vi "Write String.vi"(8 "error in (no error)":errorcluster, 9 "Colour":T1 items=["red"=0, "orange"=18, "yellow"=24, "green"=82, "cyan"=127, "blue"=170, "purple"=195, "pink"=220, "white"=254, "black"=255], 10 "String":string, 11 "Grove 2 RGB LED Matrix In":refnum<class "Grove 2 RGB LED Matrix.lvclass">) -> (0 "error out":errorcluster, 3 "Grove 2 RGB LED Matrix Out":refnum<class "Grove 2 RGB LED Matrix.lvclass">)   [LabVIEW 2020, in "CTI-Peripheral.lvlib" / "Grove 2 RGB LED Matrix.lvclass"]
uses:
  Grove 2 RGB LED Matrix.lvclass
  Data Types/Colors.ctl
  Data Types/MatrixI2CCommand.ctl
  Grove 2 RGB LED Matrix.lvclass/Grove 2 RGB LED Matrix.ctl
  CTI/I2C Connection/I2C Connection.lvclass/I2C Connection.ctl
  CTI/Session/I2C Write Data.vi
  CTI/I2C Connection/I2C Connection.lvclass
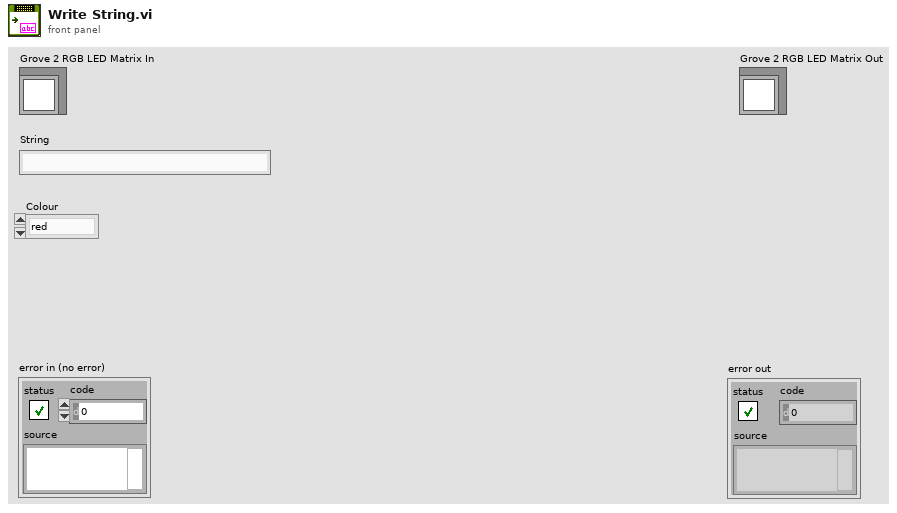
[diagram p1: front panel]
types:
  T1 = typedef "CTI-Peripheral.lvlib/Grove 2 RGB LED Matrix.lvclass/Colors.ctl" = u8
  T2 = typedef "CTI-Peripheral.lvlib/Grove 2 RGB LED Matrix.lvclass/MatrixI2CCommand.ctl" = u8
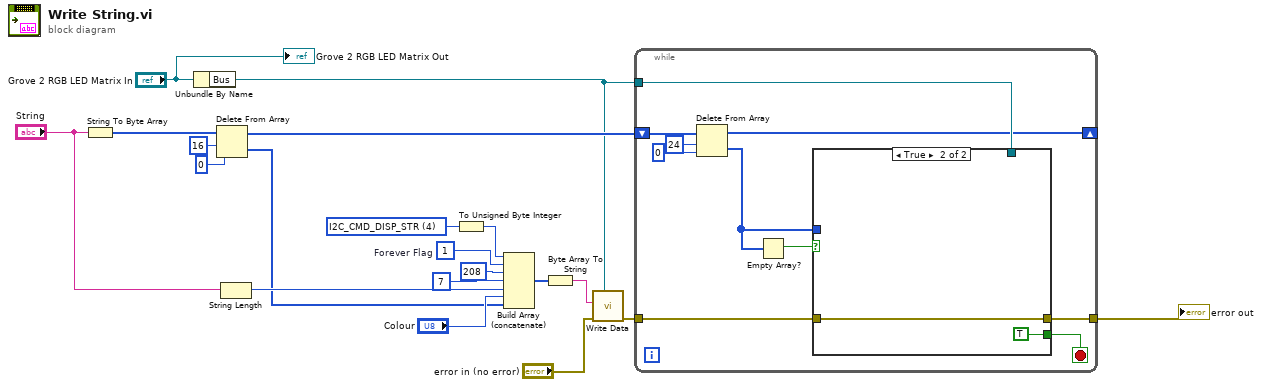
[diagram p0: block diagram]
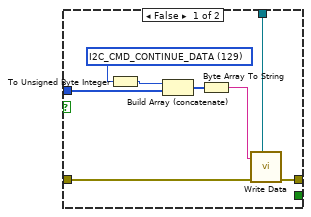
[diagram p2: hidden frame]
diagram:
  w4 = u8 1  # Forever Flag
  w9 = T2 4 items=["I2C_CMD_GET_DEV_ID"=0, "I2C_CMD_DISP_BAR"=1, "I2C_CMD_DISP_EMOJI"=2, "I2C_CMD_DISP_NUM"=3, "I2C_CMD_DISP_STR"=4, "I2C_CMD_DISP_CUSTOM"=5, "I2C_CMD_DISP_OFF"=6, "I2C_CMD_DISP_ASCII"=7, "I2C_CMD_DISP_FLASH"=8, "I2C_CMD_DISP_COLOR_BAR"=9, "I2C_CMD_DISP_COLOR_WAVE"=10, "I2C_CMD_DISP_COLOR_CLOCKWISE"=11, "I2C_CMD_DISP_COLOR_ANIMATION"=12, "I2C_CMD_DISP_COLOR_BLOCK "=13, "I2C_CMD_CONTINUE_DATA"=129, "I2C_CMD_STORE_FLASH"=160, "I2C_CMD_DELETE_FLASH"=161, "I2C_CMD_LED_ON"=176, "I2C_CMD_LED_OFF"=177, "I2C_CMD_AUTO_SLEEP_ON"=178, "I2C_CMD_AUTO_SLEEP_OFF"=179, "I2C_CMD_DISP_ROTATE"=180, "I2C_CMD_DISP_OFFSET"=181, "I2C_CMD_SET_ADDR"=192, "I2C_CMD_RST_ADDR"=193, "I2C_CMD_TEST_GET_VER"=226, "I2C_CMD_GET_DEVICE_UID"=241] ("I2C Command")
  n1 = String To Byte Array(string="String") -> (unsigned byte array=w8:u8[])
  n2 = Unbundle By Name("Grove 2 RGB LED Matrix In") -> ("Bus"=w10:refnum<class "I2C Connection.lvclass">)
  n3 = Delete From Array(array=w8, length=16, index=0) -> (deleted portion=w1:u8[], array with subset deleted=w12:u8[])
  n4 = String Length(string="String") -> (length=w3:i32)
  n5 = To Unsigned Byte Integer(number=w9) -> (unsigned 8bit integer=w5:T2)
  n6 = Build Array (concatenate)(w5, w4, u8 208, u8 7, w3, "Colour", w1) -> (w19:i32[])
  n7 = Byte Array To String(unsigned byte array=w19) -> (string=w18:string)
  n8 = call "Write Data.vi"("I2C Connection"=w10, "error in (no error)"="error in (no error)", "Data"=w18) -> ("error out"=w11:errorcluster)  [unwired: 8 in]
  n9 = while {
    tunnel: w11 -> [w27]
    tunnel: w10 -> [w26]
    tunnel: [w25] -> w7
    shift-right: [w24] -> _
    shift-left: w12 -> [w30]
    stop <- w21 stop-if-true
    n10 = Delete From Array(array=w30, length=24, index=0) -> (deleted portion=w23:u8[], array with subset deleted=w24:u8[])
    n11 = Empty Array?(array=w23) -> (empty?=w22:bool)
    n12 = case shown="True" w22 {
      tunnel: w27 -> [w36 w40]
      tunnel: w26 -> [w35 _]
      tunnel: [w32 w40] -> w25
      tunnel: w23 -> [w31 _]
      tunnel: [_ TRUE] -> w21
      frame False {
        w34 = T2 129 items=["I2C_CMD_GET_DEV_ID"=0, "I2C_CMD_DISP_BAR"=1, "I2C_CMD_DISP_EMOJI"=2, "I2C_CMD_DISP_NUM"=3, "I2C_CMD_DISP_STR"=4, "I2C_CMD_DISP_CUSTOM"=5, "I2C_CMD_DISP_OFF"=6, "I2C_CMD_DISP_ASCII"=7, "I2C_CMD_DISP_FLASH"=8, "I2C_CMD_DISP_COLOR_BAR"=9, "I2C_CMD_DISP_COLOR_WAVE"=10, "I2C_CMD_DISP_COLOR_CLOCKWISE"=11, "I2C_CMD_DISP_COLOR_ANIMATION"=12, "I2C_CMD_DISP_COLOR_BLOCK "=13, "I2C_CMD_CONTINUE_DATA"=129, "I2C_CMD_STORE_FLASH"=160, "I2C_CMD_DELETE_FLASH"=161, "I2C_CMD_LED_ON"=176, "I2C_CMD_LED_OFF"=177, "I2C_CMD_AUTO_SLEEP_ON"=178, "I2C_CMD_AUTO_SLEEP_OFF"=179, "I2C_CMD_DISP_ROTATE"=180, "I2C_CMD_DISP_OFFSET"=181, "I2C_CMD_SET_ADDR"=192, "I2C_CMD_RST_ADDR"=193, "I2C_CMD_TEST_GET_VER"=226, "I2C_CMD_GET_DEVICE_UID"=241] ("I2C Command")
        n13 = To Unsigned Byte Integer(number=w34) -> (unsigned 8bit integer=w33:T2)
        n14 = Build Array (concatenate)(w33, w31) -> (w37:T2[])
        n15 = Byte Array To String(unsigned byte array=w37) -> (string=w38:string)
        n16 = call "Write Data.vi"("I2C Connection"=w35, "error in (no error)"=w36, "Data"=w38) -> ("error out"=w32:errorcluster)  [unwired: 8 in]
      }
      frame True {
      }
    }
  }
  "error out" <- w7
  "Grove 2 RGB LED Matrix Out" <- "Grove 2 RGB LED Matrix In"
